vi "LvMPDC_SUB_ParseReplyString_Playlist.vi"(10 "string":string) -> (2 "playlist path[]":path[](array[path]))   [LabVIEW 2012]
panel:
  # "0:file: musiclibrary/BlueOysterCult/BurninForYou.mp3\nもしかしたら、file: 以外にsmb: :などの種類があるかも。"
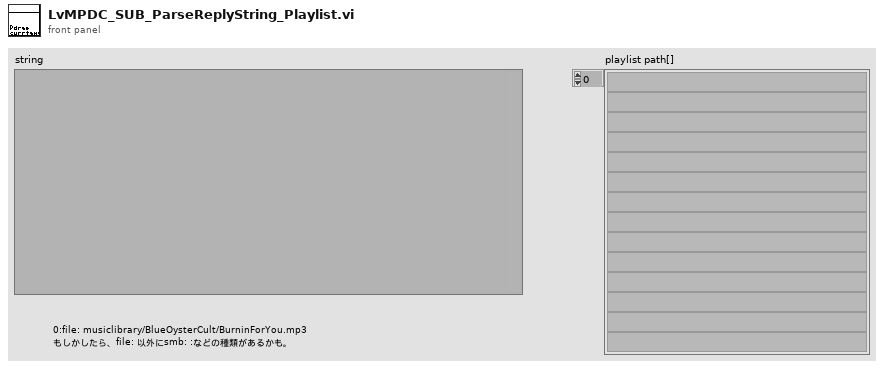
[diagram p1: front panel]
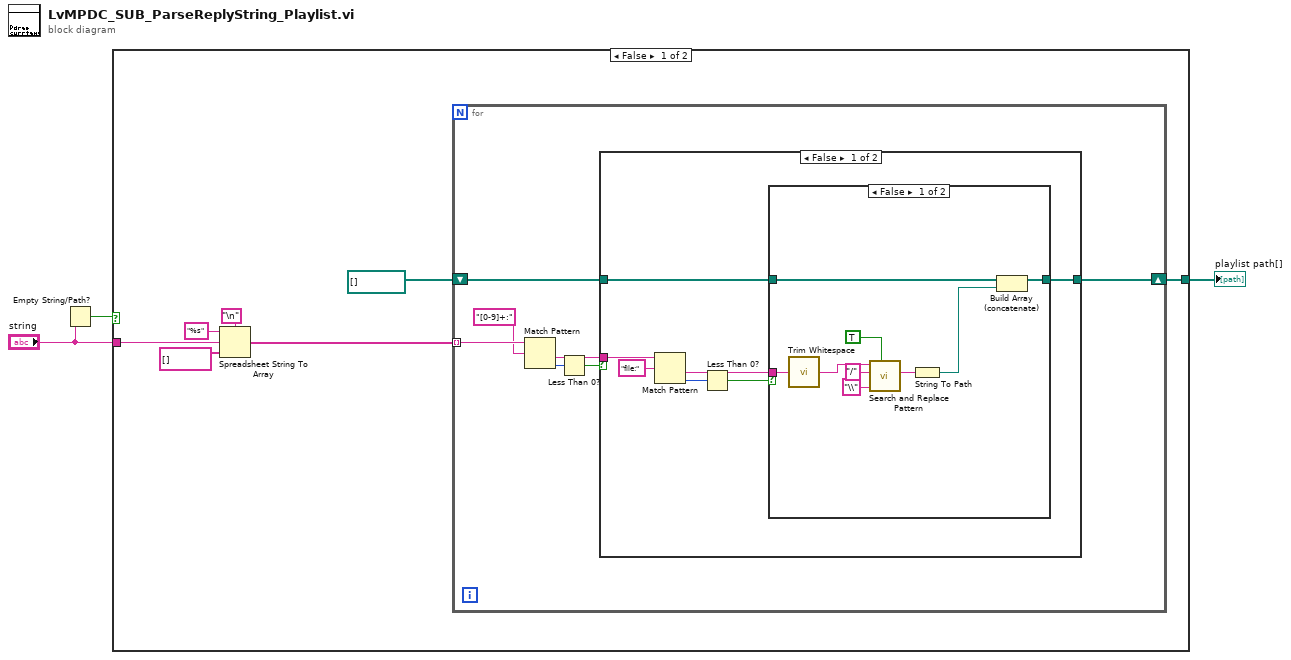
[diagram p0: block diagram]
diagram:
  n1 = Empty String/Path?(string/path="string") -> (empty?=w2:bool)
  n2 = case shown="FALSE" w2 {
    tunnel: "string" -> [w7 _]
    tunnel: [w5 _] -> w1
    frame False {
      n3 = Spreadsheet String To Array(delimiter (Tab)="\n", format string="%s" ("形式文字列"), spreadsheet string=w7, array type (2D Dbl)=string[] []) -> (array=w6:string[])
      n4 = for {
        tunnel: w6 -> [w17] mode=indexing
        shift-right: [w11] -> w5
        shift-left: path[] [] ("playlist path[]") -> [w12]
        n5 = Match Pattern(string=w17, regular expression="[0-9]+:" ("正規表現")) -> (after substring=w15:string, offset past match=w14:i32)  [unwired: 1 in, 2 out]
        n6 = Less Than 0?(x=w14) -> (x < 0?=w13:bool)
        n7 = case shown="FALSE" w13 {
          tunnel: w15 -> [w24 _]
          tunnel: w12 -> [w19 w35]
          tunnel: [w18 w35] -> w11
          frame False {
            n8 = Match Pattern(string=w24, regular expression="file:" ("正規表現")) -> (after substring=w20:string, offset past match=w22:i32)  [unwired: 1 in, 2 out]
            n9 = Less Than 0?(x=w22) -> (x < 0?=w21:bool)
            n10 = case shown="FALSE" w21 {
              tunnel: w20 -> [w31 _]
              tunnel: w19 -> [w32 w34]
              tunnel: [w33 w34] -> w18
              frame False {
                n11 = call <vilib>:"Trim Whitespace.vi"("string"=w31) -> ("trimmed string"=w29:string)  [unwired: 1 in]
                n12 = call <vilib>:"Search and Replace Pattern.vi"("string"=w29, "regular expression (\"\")"="/" ("regular expression (\"\")"), "replace string (\"\")"="\\" ("replace string (\"\")"), "replace all? (F)"=TRUE) -> ("result string"=w30:string)  [unwired: 1 in, 1 out]
                n13 = String To Path(string=w30) -> (path=w26:path)
                n14 = Build Array (concatenate)(w32, w26) -> (w33:path[])
              }
              frame True {
              }
            }
          }
          frame True {
          }
        }
      }
    }
    frame True {
    }
  }
  "playlist path[]" <- w1
